vi "Continue Waiting or Abort Dialog.vi"(8 "error in (no error)":errorcluster) -> (0 "error out":errorcluster, 3 "Abort?":bool)   [LabVIEW 2020, in "RxnRover.lvlib" / "Generic Plugin.lvclass"]
doc: "Open a dialog asking whether to continue waiting or abort the plugin."
uses:
  Generic Plugin.lvclass
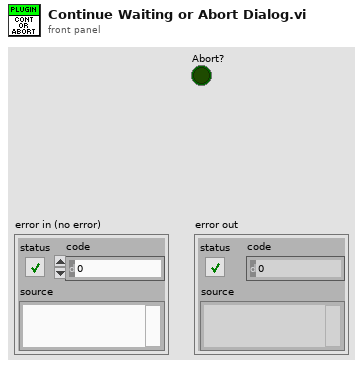
[diagram p1: front panel]
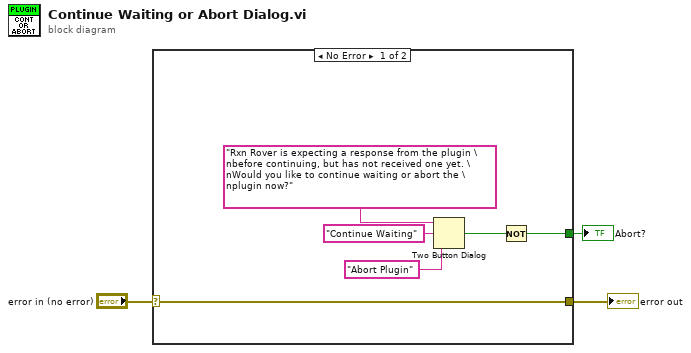
[diagram p0: block diagram]
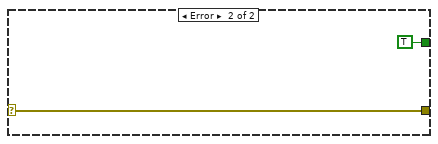
[diagram p2: hidden frame]
diagram:
  n1 = case shown="No Error" "error in (no error)" {
    selector: "error in (no error)" -> [w5 w11]
    tunnel: [w4 TRUE ("T button?")] -> w1
    tunnel: [w5 w11] -> w2
    frame No Error {
      n2 = Two Button Dialog(message="Rxn Rover is expecting a response from the plugin \nbefore continuing, but has not received one yet. \nWould you like to continue waiting or abort the \nplugin now?", 1:"Abort Plugin" ("F button name (\"Cancel\")"), 2:"Continue Waiting" ("T button name (\"OK\")")) -> (T button?=w6:bool)
      n3 = Not(x=w6) -> (.not. x?=w4:bool)
    }
    frame Error {
    }
  }
  "error out" <- w2
  "Abort?" <- w1
